vi "XLP80_TREE.vi"() -> ()   [LabVIEW 2021]
uses:
  XLP80_ProjectLibs/XLP80_Globals/Globals_Settings_XLP80.vi
panel:
  in  "Top-level VI path":path
  # "XLP80 Project\nTREE\n\n1886\n(c) 20212\n\nerstellt: \nA.Wais\nwww.m-a-r-s.de"
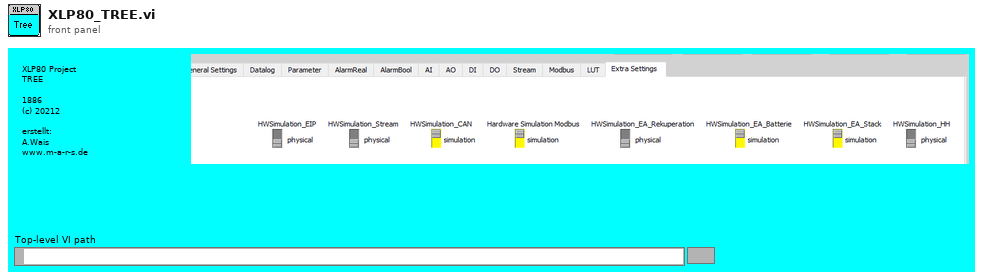
[diagram p1: front panel]
types:
  T1 = enum32{"General Settings", "Datalog", "Parameter", "AlarmReal", "AlarmBool", "AI", "AO", "DI", "DO", "CAN", "Extra Settings"}
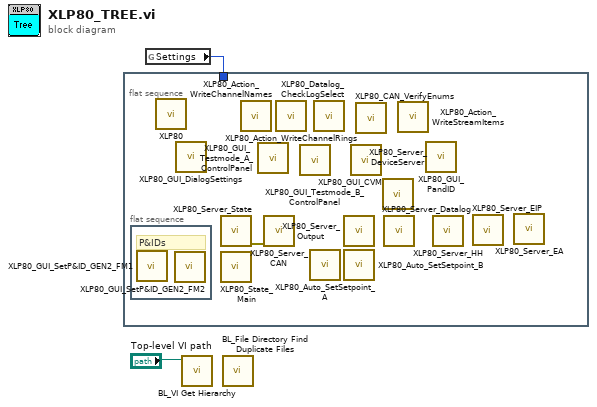
[diagram p0: block diagram]
diagram:
  n1 = flat-sequence {
    tunnel: w1 -> [_]
    frame #0 {
      n2 = flat-sequence {
        frame #0 {
          # "P&IDs"
          n3 = call "XLP80_GUI_SetP&ID_GEN2_FM1.vi"() -> ()  [unwired: 10 in, 2 out]
          n4 = call "XLP80_GUI_SetP&ID_GEN2_FM2.vi"() -> ()  [unwired: 10 in, 2 out]
        }
      }
      n5 = call "XLP80.vi"() -> ()  [unwired: 1 in]
      n6 = call "XLP80_GUI_DialogSettings.vi"() -> ()  [unwired: 10 in, 2 out]
      n7 = call "XLP80_Server_State.vi"() -> ("err out"=w3:errorcluster)  [unwired: 11 in]
      n8 = call "XLP80_State_Main.vi"() -> ()  [unwired: 11 in, 1 out]
      n9 = call "XLP80_Action_WriteChannelNames.vi"() -> ()  [unwired: 1 in]
      n10 = call "XLP80_GUI_Testmode_A_ControlPanel.vi"() -> ()  [unwired: 10 in, 2 out]
      n11 = call "XLP80_Server_CAN.vi"("err in"=w3) -> ()  [unwired: 10 in, 1 out]
      n12 = call "XLP80_Action_WriteChannelRings.vi"() -> ()  [unwired: 1 in]
      n13 = call "XLP80_GUI_Testmode_B_ControlPanel.vi"() -> ()  [unwired: 10 in, 2 out]
      n14 = call "XLP80_Auto_SetSetpoint_A.vi"() -> ()  [unwired: 11 in, 1 out]
      n15 = call "XLP80_Datalog_CheckLogSelect.vi"() -> ()  [unwired: 11 in, 1 out]
      n16 = call "XLP80_Server_Output.vi"() -> ()  [unwired: 11 in, 1 out]
      n17 = call "XLP80_Auto_SetSetpoint_B.vi"() -> ()  [unwired: 11 in, 1 out]
      n18 = call "XLP80_GUI_CVM.vi"() -> ()  [unwired: 11 in, 1 out]
      n19 = call "XLP80_CAN_VerifyEnums.vi"() -> ()  [unwired: 11 in, 1 out]
      n20 = call "XLP80_Server_DeviceServer.vi"() -> ()  [unwired: 11 in, 1 out]
      n21 = call "XLP80_Server_Datalog.vi"() -> ()  [unwired: 11 in, 1 out]
      n22 = call "XLP80_Action_WriteStreamItems.vi"() -> ()  [unwired: 11 in, 1 out]
      n23 = call "XLP80_GUI_PandID.vi"() -> ()  [unwired: 11 in, 1 out]
      n24 = call "XLP80_Server_HH.vi"() -> ()  [unwired: 11 in, 1 out]
      n25 = call "XLP80_Server_EIP.vi"() -> ()  [unwired: 11 in, 1 out]
      n26 = call "XLP80_Server_EA.vi"() -> ()  [unwired: 11 in, 1 out]
    }
  }
  n27 = global read "Globals_Settings_XLP80.vi" "Settings"() -> (w1:T1)
  n28 = call "BL_VI Get Hierarchy.vi"("Top-level VI path"="Top-level VI path") -> ()  [unwired: 7 in, 4 out]
  n29 = call "BL_File Directory Find Duplicate Files.vi"() -> ()  [unwired: 8 in, 4 out]
